vi "Configure Buffer Storage.vi"(0 "VISA resource name":refnum<visa-resource-name>, 1 "Number of Points (2)":dbl=2.0 min=2.0 max=2000.0 step=1.0 format="%#.0f", 5 "Storage Type (2:All)":u16(ring)=2 items=["Voltage", "Current", "All"], 7 "Trigger Delay (0)":dbl min=0.0 max=3600.0 step=0.01 format="%#.2f", 9 "Time Interval (1)":dbl=1.0 min=0.0002 max=3600.0 step=1.0 format="%#_4f", 11 "error in (no error)":errorcluster, 12 "Enable Filter (F: False)":bool, 13 "Clear Buffer? (T: True)":bool=TRUE) -> (4 "VISA resource name out":refnum<visa-resource-name>, 15 "error out":errorcluster)   [LabVIEW 2018, in "BK Precision 8600 Series.lvlib"]
doc: "Configures the instrument for buffer storage operation. This VI allows the instrument to store a specified number of points that contain measured voltage, current, or both readings (it will be half the number of points specified) into internal buffer, which can later be retrieved using <b>Read Buffer Data.vi</b>.\n\nIt is recommended to clear all buffer data first before configuring this operation.\n\nNote: Trigger should be setup prior to configuring for buffer storage operation using <b>Configure Trigger.vi</b>.\n\nA trigger must be received to initiate buffer storage operation. Use <b>Enable Buffer Storage.vi</b> after this vi to begin the storage operation."
uses:
  <instrlib>/BK Precision 8600 Series/BK Precision 8600 Series.lvlib
panel:
  # "s"
  # "s"
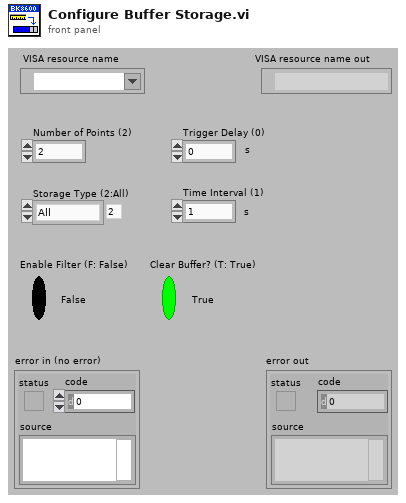
[diagram p1: front panel]
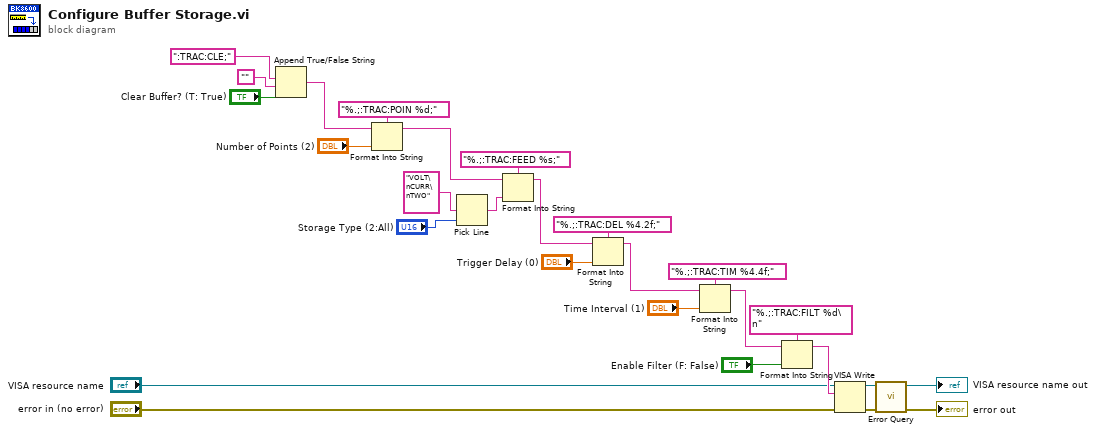
[diagram p0: block diagram]
diagram:
  n1 = Append True/False String(1:"Clear Buffer? (T: True)", 2:"", 3:":TRAC:CLE;") -> (0:w21:string)  [unwired: 1 in]
  n2 = Format Into String(format string="%.;:TRAC:POIN %d;", initial string=w21, "Number of Points (2)") -> (resulting string=w15:string)  [unwired: 1 in, 1 out]
  n3 = Pick Line(multi-line string="VOLT\nCURR\nTWO", line index="Storage Type (2:All)") -> (output string=w16:string)  [unwired: 1 in]
  n4 = Format Into String(format string="%.;:TRAC:FEED %s;", initial string=w15, w16) -> (resulting string=w14:string)  [unwired: 1 in, 1 out]
  n5 = Format Into String(format string="%.;:TRAC:DEL %4.2f;", initial string=w14, "Trigger Delay (0)") -> (resulting string=w11:string)  [unwired: 1 in, 1 out]
  n6 = Format Into String(format string="%.;:TRAC:TIM %4.4f;", initial string=w11, "Time Interval (1)") -> (resulting string=w8:string)  [unwired: 1 in, 1 out]
  n7 = Format Into String(format string="%.;:TRAC:FILT %d\n", initial string=w8, "Enable Filter (F: False)") -> (resulting string=w3:string)  [unwired: 1 in, 1 out]
  n8 = VISA Write(VISA resource name="VISA resource name", write buffer=w3, error in (no error)="error in (no error)") -> (VISA resource name out=w7:refnum<visa-resource-name>, error out=w6:errorcluster)  [unwired: 1 out]
  n9 = call <instrlib>:"Error Query.vi"("error in (no error)"=w6, "VISA resource name"=w7) -> ("error out"=→"error out":errorcluster, "VISA resource name out"=→"VISA resource name out":refnum<visa-resource-name>)  [unwired: 6 in, 2 out]
